vi "get_value_for_integer.vi"(8 "error in (no error)":errorcluster, 11 "Value in":refnum<class "Value.lvclass">) -> (0 "error out":errorcluster, 2 "integer_value":i64, 3 "Value out":refnum<class "Value.lvclass">)   [LabVIEW 2020, in "toml_edit.lvlib" / "Value.lvclass"]
uses:
  Value.lvclass
  Value.lvclass/Value.ctl
  dragon_toml_64.dll
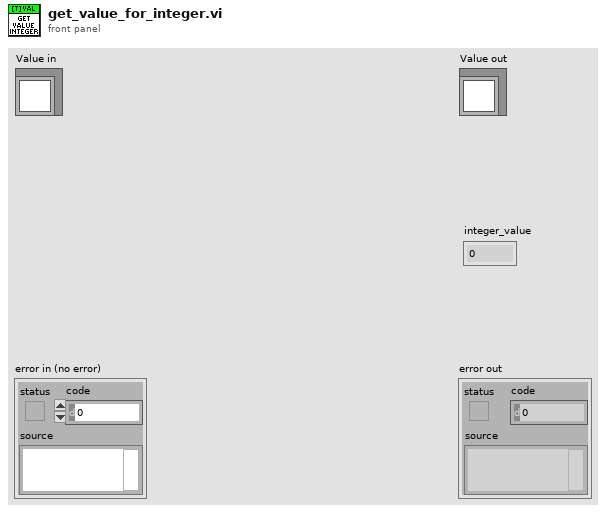
[diagram p1: front panel]
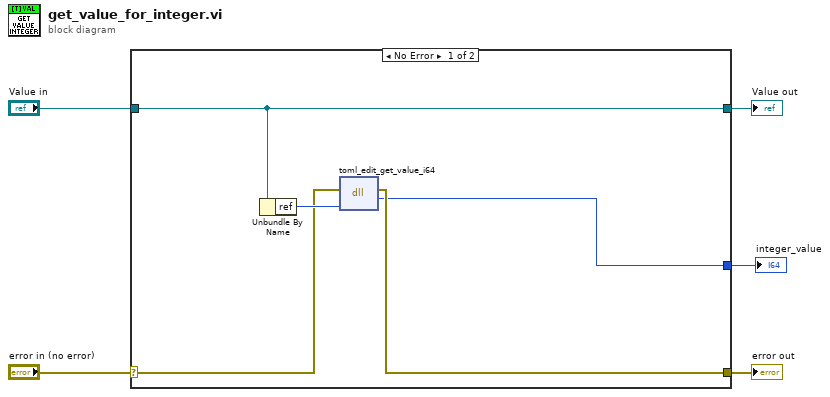
[diagram p0: block diagram]
diagram:
  n1 = case shown="No Error" "error in (no error)" {
    selector: "error in (no error)" -> [w7 w12]
    tunnel: [w10 w12] -> w4
    tunnel: [w8 w11] -> w2
    tunnel: "Value in" -> [w8 w11]
    tunnel: [w6 _] -> w1
    frame No Error {
      n2 = Unbundle By Name(w8) -> ("ref"=w9:u64)
      n3 = dll-call lib="C:/Projects/toml-edit-labview/lv_src/dragon_toml_*.dll" fn="toml_edit_get_value_i64"(error in=w7, "item"=w9) -> (error out=w10:errorcluster, "i64_value"=w6:i64)  [unwired: 3 in, 1 out]
    }
    frame Error {
    }
  }
  "error out" <- w4
  "Value out" <- w2
  "integer_value" <- w1
